vi "calExport.vi"(5 "date/time string":string, 8 "error in (no error)":errorcluster, 9 "660 Calibration":T1, 10 "532 Calibration":T1) -> (0 "error out":errorcluster)   [LabVIEW 2011]
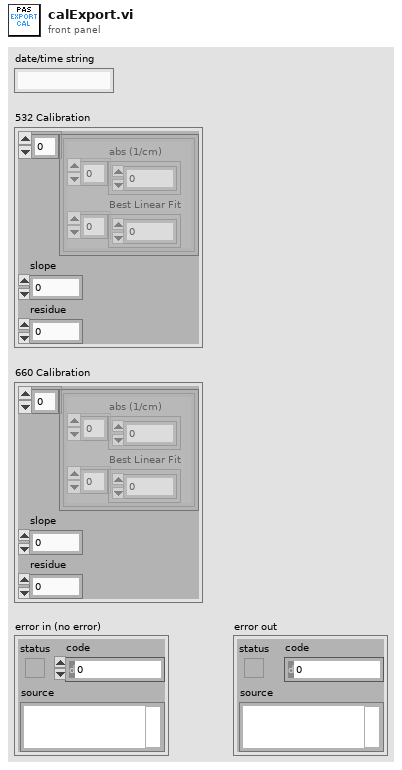
[diagram p1: front panel]
types:
  T1 = cluster{cluster{"abs (1/cm)":dbl[], "Best Linear Fit":dbl[]}[], "slope":dbl, "residue":dbl}
  T2 = cluster{"abs (1/cm)":dbl[], "Best Linear Fit":dbl[]}[]
  T3 = cluster{"abs (1/cm)":dbl[], "Best Linear Fit":dbl[]}
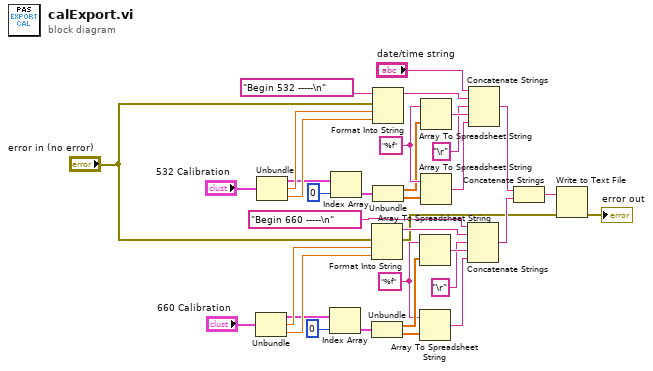
[diagram p0: block diagram]
diagram:
  w23 = "%f" ("format string")
  w22 = "%f" ("format string")
  n1 = Unbundle("660 Calibration") -> (w25:T2, "slope"=w34:dbl, "residue"=w35:dbl)
  n2 = Unbundle("532 Calibration") -> (w16:T2, "slope"=w17:dbl, "residue"=w18:dbl)
  n3 = Index Array(array=w25, index=0) -> (element=w28:T3)
  n4 = Index Array(array=w16, index=0) -> (element=w15:T3)
  n5 = Format Into String(error in="error in (no error)", w34, w35) -> (resulting string=w24:string, error out=w11:errorcluster)  [unwired: 2 in]
  n6 = Unbundle(w28) -> ("abs (1/cm)"=w29:dbl[], "Best Linear Fit"=w30:dbl[])
  n7 = Format Into String(initial string="Begin 532 -----\n" ("string"), error in="error in (no error)", w17, w18) -> (resulting string=w21:string)  [unwired: 1 in, 1 out]
  n8 = Unbundle(w15) -> ("abs (1/cm)"=w19:dbl[], "Best Linear Fit"=w20:dbl[])
  n9 = Array To Spreadsheet String(array=w29, 3:w23) -> (spreadsheet string=w7:string)  [unwired: 1 in]
  n10 = Array To Spreadsheet String(array=w30, 3:w23) -> (spreadsheet string=w4:string)  [unwired: 1 in]
  n11 = Array To Spreadsheet String(array=w19, 3:w22) -> (spreadsheet string=w9:string)  [unwired: 1 in]
  n12 = Array To Spreadsheet String(array=w20, 3:w22) -> (spreadsheet string=w5:string)  [unwired: 1 in]
  n13 = Concatenate Strings("Begin 660 -----\n" ("string"), w24, "\r" ("string"), w7, w4) -> (w33:string)
  n14 = Concatenate Strings("date/time string", w21, "\r" ("string"), w9, w5) -> (w32:string)
  n15 = Concatenate Strings(w32, w33) -> (w12:string)
  n16 = Write to Text File(text=w12, error in=w11) -> (error out=→"error out":errorcluster)  [unwired: 2 in, 2 out]
